vi "Close.vi"(8 "error in (no error)":errorcluster, 11 "SimPID in":refnum<class "SimPID.lvclass">) -> (0 "error out":errorcluster, 3 "SimPID out":refnum<class "SimPID.lvclass">)   [LabVIEW 2023, in "SimPID.lvclass"]
uses:
  SimPID.lvclass
  SimPID.lvclass/SimPID.ctl
  PIDController/PIDController.lvclass
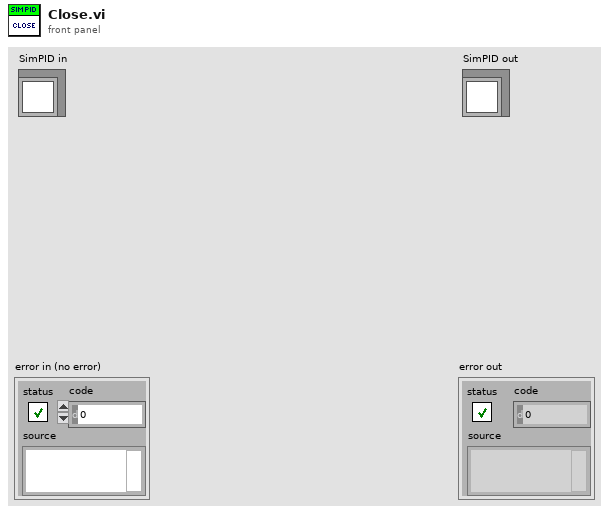
[diagram p1: front panel]
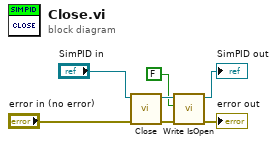
[diagram p0: block diagram]
diagram:
  n1 = call-parent "Close.vi"("error in (no error)"="error in (no error)", "PIDController in"="SimPID in") -> ("error out"=w3:errorcluster, "PIDController out"=w5:refnum<class "SimPID.lvclass">)  [unwired: 8 in]
  n2 = call-dynamic "Write IsOpen.vi"("error in (no error)"=w3, "IsOpen"=FALSE, "PIDController in"=w5) -> ("error out"=→"error out":errorcluster, "PIDController out"=→"SimPID out":refnum<class "SimPID.lvclass">)  [unwired: 7 in]
